vi "extractTopicContents.vi"(8 "error in (no error)":errorcluster, 10 "topicName":string, 11 "Module in":refnum<class "Module.lvclass">) -> (0 "error out":errorcluster, 2 "topicContentsString":string, 3 "Module out":refnum<class "Module.lvclass">)   [LabVIEW 2016, in "Module.lvclass"]
uses:
  Module.lvclass
  Module.lvclass/Module.ctl
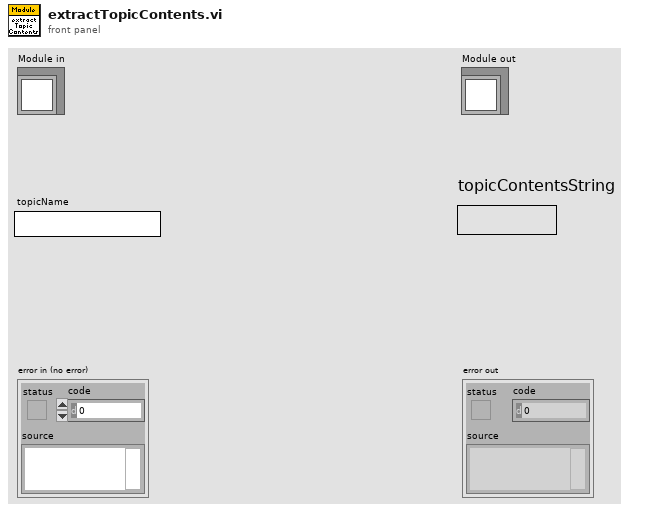
[diagram p1: front panel]
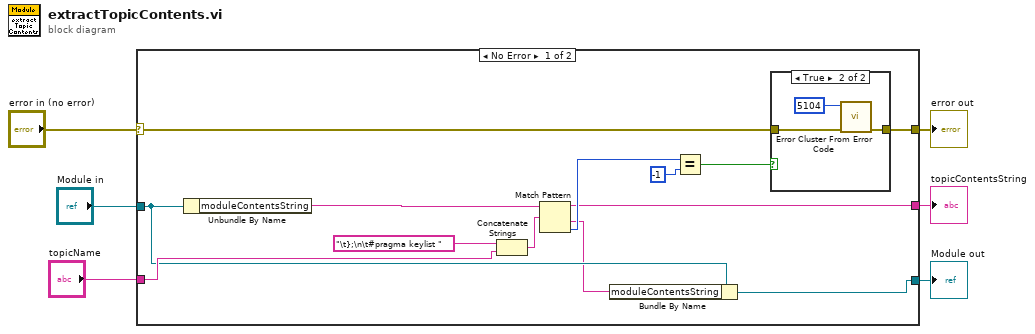
[diagram p0: block diagram]
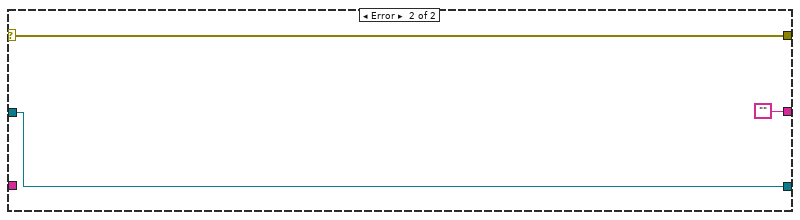
[diagram p3: hidden frame]
diagram:
  n1 = case shown="No Error" "error in (no error)" {
    selector: "error in (no error)" -> [w8 w26]
    tunnel: [w7 w26] -> w5
    tunnel: [w12 w25] -> w3
    tunnel: "Module in" -> [w13 w25]
    tunnel: "topicName" -> [w14 _]
    tunnel: [w10 ""] -> w1
    frame No Error {
      n2 = Unbundle By Name(w13) -> ("moduleContentsString"=w15:string)
      n3 = Concatenate Strings("\t};\n\t#pragma keylist " ("regular expression"), w14) -> (w16:string)
      n4 = Match Pattern(string=w15, regular expression=w16) -> (before substring=w10:string, after substring=w11:string, offset past match=w18:i32)  [unwired: 1 in, 1 out]
      n5 = Bundle By Name(cluster=w13, "moduleContentsString"=w11) -> (w12:refnum<class "Module.lvclass">)
      n6 = Equal?(x=w18, y=-1) -> (x = y?=w9:bool)
      n7 = case shown="True" w9 {
        tunnel: w8 -> [w20 w22]
        tunnel: [w20 w21] -> w7
        frame False {
        }
        frame True {
          n8 = call <vilib>:"Error Cluster From Error Code.vi"("error in (no error)"=w22, "error code (0)"=5104) -> ("error out"=w21:errorcluster)  [unwired: 7 in]
        }
      }
    }
    frame Error {
    }
  }
  "error out" <- w5
  "Module out" <- w3
  "topicContentsString" <- w1
